vi "HFRR ADV v024 new software.vi"() -> ()   [LabVIEW 2025] (continued)
            n1309 = call "CAMERA LIVE FEED FGV.vi"("Enum - Menu"=CAMERA_LIVE_FEED_ENUM."CAMERA MINIMIZE") -> ()  [unwired: 9 in, 2 out]
          }
          frame #1 {
            n1310 = property on="Auto Scar Check  2" class="Clust (strict)"("Visible"=TRUE) -> ()  [unwired: 2 in, 2 out]
          }
          frame #2 {
            n1311 = String To Path(string="C:\\LAB-IQ\\Image Calibrate v01.dcf") -> (path=w1382:path)
            n1312 = Open/Create/Replace File ("Open File")(file path (use dialog)=w1382) -> (refnum out=w1383:refnum<file>)  [unwired: 5 in, 2 out]
            n1313 = for {
              N: 4 -> [_]
              tunnel: w1383 -> [w1389]
              i -> [w1385]
              n1314 = Read from Text File ("Read File")(file (use dialog)=w1389) -> (text=w1390:string)  [unwired: 3 in, 3 out]
              n1315 = String Subset(string=w1390, offset (0)=6, length (rest)=10 ("length (rest)")) -> (substring=w1386:string)
              n1316 = Fract/Exp String To Number(string=w1386) -> (number=w1384:dbl)  [unwired: 3 in, 1 out]
              n1317 = case shown="0" w1385 {
                tunnel: w1384 -> [w1391 w1392 _ w1393 _]
                frame 0 {
                  "5x Gain" <- w1391
                }
                frame 1 {
                  "10x Gain" <- w1392
                }
                frame 2 {
                }
                frame 3 {
                  "100x gain" <- w1393
                }
                frame 4, Default {
                }
              }
            }
          }
          frame #3 {
            n1318 = local read "FILE 3"() -> (w1399:string)
            n1319 = call <vilib>:"Trim Whitespace.vi"("string"="C:\\LAB-IQ\\images\\") -> ("trimmed string"=w1401:string)  [unwired: 1 in]
            n1320 = String To Path(string=w1401) -> (path=w1400:path)
            n1321 = Concatenate Strings(w1399, ".png" ("string")) -> (w1398:string)
            n1322 = Build Path(base path=w1400, name or relative path=w1398) -> (appended path=w1396:path)
            "Image path" <- w1396
            n1323 = Path To String(path=w1396) -> (string=w1395:string)
            n1324 = call "CAMERA LIVE FEED FGV.vi"("Enum - Menu"=CAMERA_LIVE_FEED_ENUM."CAMERA SAVE", "Image Path"=w1395) -> ()  [unwired: 8 in, 2 out]
          }
          frame #4 {
            n1325 = One Button Dialog(message="Image saved successfully") -> ()  [unwired: 1 in, 1 out]
          }
          frame #5 {
            n1326 = local read "TEST STANDARD"() -> (w1405:T3)
            n1327 = local read "Magnification len live scar"() -> (w1417:string)
            n1328 = Not(x=w1406) -> (.not. x?=w1407:bool)
            n1329 = local write "Cap Live Image"(w1407) -> ()
            n1330 = case shown="\"ISO 12156\"" w1405 {
              tunnel: ["ASTM D6079" "ISO 12156"] -> w1404
              frame "ASTM D6079", Default {
              }
              frame "ISO 12156" {
              }
            }
            n1331 = case shown="\"5x\", Default" w1417 {
              tunnel: [w1420 w1421] -> w1416
              frame "5x", Default {
                n1332 = local read "5x Gain"() -> (w1420:dbl)
              }
              frame "10x" {
                # "5x"
                n1333 = local read "10x Gain"() -> (w1421:dbl)
              }
            }
            n1334 = local read "Image path"() -> (w1415:path)
            n1335 = local read "FILE 3"() -> (w1408:string)
            n1336 = call "EDGE DETCTION.vi"("GAIN VALUE"=w1416, "Image Path"=w1415) -> ("error out"=w1414:errorcluster, "return value"=w1413:cluster{string, string, dbl, dbl, dbl})  [unwired: 8 in]
            n1337 = Bundle By Name(cluster=T25 {"File Name"="", "Test Method"="", "Operator"="", "Fuel Description"="", "Date and time"=""} ("Main Ref"), "File Name"=w1408, "Test Method"=w1404) -> (w1409:T25)
            n1338 = call "duf file read.vi"("error in (no error)"=w1414, "Main Ref"=w1409) -> ("error out"=w1412:errorcluster, "Main Ref 2"=w1410:T25)  [unwired: 8 in]
            n1339 = call "EDGE DETECTION REPORT.vi"("error in (no error)"=w1412, "return value 2"=w1413, "Main Ref"=w1410) -> ()  [unwired: 8 in, 1 out]
          }
          frame #6 {
            n1340 = property on="Auto Scar Check  2" class="Clust (strict)"("Visible"=FALSE) -> ()  [unwired: 2 in, 2 out]
          }
          frame #7 {
            n1341 = call "CAMERA LIVE FEED FGV.vi"("Enum - Menu"=CAMERA_LIVE_FEED_ENUM."CAMERA MINIMIZE", "error in (no error)"=w1425) -> ()  [unwired: 8 in, 2 out]
            n1342 = local write "Main Dashboard Buttons"(T1."Home" ("Main Dashboard Buttons")) -> ()
            n1343 = local write "Main Tab"(T2."HOME" ("Main Tab")) -> ()
          }
        }
      }
    }
    n1344 = local read "Heater Button"() -> (w1278:bool)
    n1345 = case shown="True" w1280 {
      selector: w1280 -> [_ w1555]
      frame False {
      }
      frame True {
        n1346 = Not(x=w1555) -> (.not. x?=w1553:bool)
        n1347 = local write "Frequency"(w1553) -> ()
        n1348 = local write "Tab Control 2"(T6."Frequency" ("Tab Control 2")) -> ()
      }
    }
    n1349 = case shown="True" w1279 {
      selector: w1279 -> [_ w1552]
      frame False {
      }
      frame True {
        n1350 = Not(x=w1552) -> (.not. x?=w1550:bool)
        n1351 = local write "Air Temp vs Humidity"(w1550) -> ()
        n1352 = local write "Tab Control 2"(T6."Air Temp vs Rh" ("Tab Control 2")) -> ()
      }
    }
    n1353 = case shown="True" w1281 {
      selector: w1281 -> [_ w1558]
      frame False {
      }
      frame True {
        n1354 = Not(x=w1558) -> (.not. x?=w1556:bool)
        n1355 = local write "Sample Temperature"(w1556) -> ()
        n1356 = local write "Tab Control 2"(T6."Sample Temperature" ("Tab Control 2")) -> ()
      }
    }
    n1357 = case shown="\"Custom\"" w1277 {
      frame "ASTM D6079", Default {
        w1531 = "ASTM D6079 TEST CONDITIONS" ("Standard 2")
        n1358 = local write "Standard 2"(w1531) -> ()
        n1359 = local write "Standard"(w1531) -> ()
      }
      frame "ISO 12156" {
        w1532 = "ISO 12156 TEST CONDITIONS" ("Standard 2")
        n1360 = local write "Standard 2"(w1532) -> ()
        n1361 = local write "Standard"(w1532) -> ()
      }
      frame "CEC F-096-A-06" {
        w1533 = "CEC F-096-A-06 TEST CONDITIONS" ("Standard 2")
        n1362 = local write "Standard 2"(w1533) -> ()
        n1363 = local write "Standard"(w1533) -> ()
      }
      frame "Custom" {
        w1534 = "CUSTOM TEST CONDITIONS" ("Standard 2")
        n1364 = local write "Standard 2"(w1534) -> ()
        n1365 = local write "Standard"(w1534) -> ()
      }
    }
    n1366 = case shown="True" w1278 {
      frame False {
        n1367 = local write "Temperature On Command"(TRUE ("Temperature On Command")) -> ()
        n1368 = case shown="True" "Temperature Off Command" {
          selector: "Temperature Off Command" -> [_ w1538]
          frame False {
          }
          frame True {
            n1369 = Not(x=w1538) -> (.not. x?=w1537:bool)
            n1370 = local read "EVENT LOG"() -> (w1541:string)
            n1371 = local write "Temperature Off Command"(w1537) -> ()
            n1372 = call "Event Log.vi"("Content"="Heater Off", "EVENT LOG"=w1541) -> ("EVENT LOG"=w1540:string)  [unwired: 8 in, 1 out]
            n1373 = local write "EVENT LOG"(w1540) -> ()
          }
        }
      }
      frame True {
        n1374 = local write "Temperature Off Command"(TRUE ("Temperature Off Command")) -> ()
        n1375 = case shown="True" "Temperature On Command" {
          selector: "Temperature On Command" -> [_ w1545]
          frame False {
          }
          frame True {
            n1376 = Not(x=w1545) -> (.not. x?=w1544:bool)
            n1377 = local write "Temperature On Command"(w1544) -> ()
            n1378 = disable-structure shown="Enabled" {
              disable-tunnel: "Heater On" -> [w1547 _]
              frame Enabled {
                n1379 = local read "EVENT LOG"() -> (w1548:string)
                n1380 = call "Event Log.vi"("Content"=w1547, "EVENT LOG"=w1548) -> ("EVENT LOG"=w1549:string)  [unwired: 8 in, 1 out]
                n1381 = local write "EVENT LOG"(w1549) -> ()
              }
              frame Disabled {
              }
            }
          }
        }
      }
    }
    n1382 = local read "Main Tab"() -> (w1269:T2)
    n1383 = case shown="\"About\"" w1269 {
      frame "HOME", Default {
        w1312 = T19."Enabled" ("Disabled")
        n1384 = local read "Service Password enable"() -> (w1314:bool)
        n1385 = property on="Imaging" class="Bool (strict)"("DisabledEnum"=w1312) -> ()  [unwired: 2 in, 2 out]
        n1386 = property on="Dashboard" class="Bool (strict)"("DisabledEnum"=w1312) -> ()  [unwired: 2 in, 2 out]
        n1387 = property on="Test Setup" class="Bool (strict)"("DisabledEnum"=w1312) -> ()  [unwired: 2 in, 2 out]
        n1388 = property on="Analysis" class="Bool (strict)"("DisabledEnum"=w1312) -> ()  [unwired: 2 in, 2 out]
        n1389 = property on="Home" class="Bool (strict)"("DisabledEnum"=w1312) -> ()  [unwired: 2 in, 2 out]
        n1390 = property on="Report" class="Bool (strict)"("DisabledEnum"=w1312) -> ()  [unwired: 2 in, 2 out]
        n1391 = property on="Main Dashboard Buttons" class="RadioBtnsControl (strict)"("DisabledEnum"=w1312) -> ()  [unwired: 2 in, 2 out]
        n1392 = property on="Calibration" class="Bool (strict)"("DisabledEnum"=w1312) -> ()  [unwired: 2 in, 2 out]
        n1393 = case shown="True" w1314 {
          tunnel: [T19."Disabled" ("Disabled") T19."Enabled" ("Disabled")] -> w1313
          frame False {
          }
          frame True {
          }
        }
        n1394 = property on="About" class="Bool (strict)"("DisabledEnum"=w1313) -> ()  [unwired: 2 in, 2 out]
      }
      frame "Test Setup" {
        w1319 = T19."Enabled" ("Disabled")
        n1395 = local read "Service Password enable"() -> (w1318:bool)
        n1396 = property on="Dashboard" class="Bool (strict)"("DisabledEnum"=T19."Disabled" ("Disabled")) -> ()  [unwired: 2 in, 2 out]
        n1397 = property on="Imaging" class="Bool (strict)"("DisabledEnum"=w1319) -> ()  [unwired: 2 in, 2 out]
        n1398 = property on="Analysis" class="Bool (strict)"("DisabledEnum"=w1319) -> ()  [unwired: 2 in, 2 out]
        n1399 = property on="Home" class="Bool (strict)"("DisabledEnum"=w1319) -> ()  [unwired: 2 in, 2 out]
        n1400 = property on="Report" class="Bool (strict)"("DisabledEnum"=w1319) -> ()  [unwired: 2 in, 2 out]
        n1401 = property on="Test Setup" class="Bool (strict)"("DisabledEnum"=w1319) -> ()  [unwired: 2 in, 2 out]
        n1402 = case shown="True" w1318 {
          tunnel: [T19."Disabled" ("Disabled") T19."Enabled" ("Disabled")] -> w1317
          frame False {
          }
          frame True {
          }
        }
        n1403 = property on="About" class="Bool (strict)"("DisabledEnum"=w1317) -> ()  [unwired: 2 in, 2 out]
      }
      frame "Adv Scar" {
        w1326 = T19."Enabled" ("Disabled")
        n1404 = property on="Dashboard" class="Bool (strict)"("DisabledEnum"=T19."Disabled" ("Disabled")) -> ()  [unwired: 2 in, 2 out]
        n1405 = property on="Imaging" class="Bool (strict)"("DisabledEnum"=w1326) -> ()  [unwired: 2 in, 2 out]
        n1406 = property on="Analysis" class="Bool (strict)"("DisabledEnum"=w1326) -> ()  [unwired: 2 in, 2 out]
        n1407 = property on="Home" class="Bool (strict)"("DisabledEnum"=w1326) -> ()  [unwired: 2 in, 2 out]
        n1408 = property on="Report" class="Bool (strict)"("DisabledEnum"=w1326) -> ()  [unwired: 2 in, 2 out]
        n1409 = property on="Test Setup" class="Bool (strict)"("DisabledEnum"=w1326) -> ()  [unwired: 2 in, 2 out]
        n1410 = local read "Service Password enable"() -> (w1324:bool)
        n1411 = case shown="True" w1324 {
          tunnel: [T19."Disabled" ("Disabled") T19."Enabled" ("Disabled")] -> w1323
          frame False {
          }
          frame True {
          }
        }
        n1412 = property on="About" class="Bool (strict)"("DisabledEnum"=w1323) -> ()  [unwired: 2 in, 2 out]
      }
      frame "Calibration" {
        w1329 = T19."Enabled" ("Disabled")
        n1413 = property on="Dashboard" class="Bool (strict)"("DisabledEnum"=T19."Disabled" ("Disabled")) -> ()  [unwired: 2 in, 2 out]
        n1414 = property on="Imaging" class="Bool (strict)"("DisabledEnum"=w1329) -> ()  [unwired: 2 in, 2 out]
        n1415 = property on="Analysis" class="Bool (strict)"("DisabledEnum"=w1329) -> ()  [unwired: 2 in, 2 out]
        n1416 = property on="Home" class="Bool (strict)"("DisabledEnum"=w1329) -> ()  [unwired: 2 in, 2 out]
        n1417 = property on="Report" class="Bool (strict)"("DisabledEnum"=w1329) -> ()  [unwired: 2 in, 2 out]
        n1418 = property on="Test Setup" class="Bool (strict)"("DisabledEnum"=w1329) -> ()  [unwired: 2 in, 2 out]
        n1419 = local read "Service Password enable"() -> (w1331:bool)
        n1420 = property on="Calibration" class="Bool (strict)"("DisabledEnum"=w1329) -> ()  [unwired: 2 in, 2 out]
        n1421 = case shown="True" w1331 {
          tunnel: [T19."Disabled" ("Disabled") T19."Enabled" ("Disabled")] -> w1330
          frame False {
          }
          frame True {
          }
        }
        n1422 = property on="About" class="Bool (strict)"("DisabledEnum"=w1330) -> ()  [unwired: 2 in, 2 out]
      }
      frame "Adv Scar Report" {
        w1337 = T19."Enabled" ("Disabled")
        n1423 = property on="Dashboard" class="Bool (strict)"("DisabledEnum"=T19."Disabled" ("Disabled")) -> ()  [unwired: 2 in, 2 out]
        n1424 = property on="Imaging" class="Bool (strict)"("DisabledEnum"=w1337) -> ()  [unwired: 2 in, 2 out]
        n1425 = property on="Analysis" class="Bool (strict)"("DisabledEnum"=w1337) -> ()  [unwired: 2 in, 2 out]
        n1426 = property on="Home" class="Bool (strict)"("DisabledEnum"=w1337) -> ()  [unwired: 2 in, 2 out]
        n1427 = property on="Report" class="Bool (strict)"("DisabledEnum"=w1337) -> ()  [unwired: 2 in, 2 out]
        n1428 = property on="Test Setup" class="Bool (strict)"("DisabledEnum"=w1337) -> ()  [unwired: 2 in, 2 out]
        n1429 = local read "Service Password enable"() -> (w1336:bool)
        n1430 = case shown="True" w1336 {
          tunnel: [T19."Disabled" ("Disabled") T19."Enabled" ("Disabled")] -> w1335
          frame False {
          }
          frame True {
          }
        }
        n1431 = property on="About" class="Bool (strict)"("DisabledEnum"=w1335) -> ()  [unwired: 2 in, 2 out]
      }
      frame "Compare Files" {
        w1343 = T19."Enabled" ("Disabled")
        n1432 = local read "Service Password enable"() -> (w1342:bool)
        n1433 = property on="Dashboard" class="Bool (strict)"("DisabledEnum"=T19."Disabled" ("Disabled")) -> ()  [unwired: 2 in, 2 out]
        n1434 = property on="Imaging" class="Bool (strict)"("DisabledEnum"=w1343) -> ()  [unwired: 2 in, 2 out]
        n1435 = property on="Analysis" class="Bool (strict)"("DisabledEnum"=w1343) -> ()  [unwired: 2 in, 2 out]
        n1436 = property on="Home" class="Bool (strict)"("DisabledEnum"=w1343) -> ()  [unwired: 2 in, 2 out]
        n1437 = property on="Report" class="Bool (strict)"("DisabledEnum"=w1343) -> ()  [unwired: 2 in, 2 out]
        n1438 = property on="Test Setup" class="Bool (strict)"("DisabledEnum"=w1343) -> ()  [unwired: 2 in, 2 out]
        n1439 = case shown="True" w1342 {
          tunnel: [T19."Disabled" ("Disabled") T19."Enabled" ("Disabled")] -> w1341
          frame False {
          }
          frame True {
          }
        }
        n1440 = property on="About" class="Bool (strict)"("DisabledEnum"=w1341) -> ()  [unwired: 2 in, 2 out]
      }
      frame "Acquire" {
        n1441 = local read "Service Password enable"() -> (w1348:bool)
        n1442 = property on="Test Setup" class="Bool (strict)"("DisabledEnum"=T19."Disabled" ("Disabled")) -> ()  [unwired: 2 in, 2 out]
        n1443 = local read "Auto Start Test"() -> (w1350:bool)
        n1444 = local read "RUN"() -> (w1352:bool)
        n1445 = case shown="True" w1348 {
          tunnel: [T19."Disabled" ("Disabled") T19."Enabled" ("Disabled")] -> w1349
          frame False {
          }
          frame True {
          }
        }
        n1446 = Or(x=w1352, y=w1350) -> (x .or. y?=w1351:bool)
        n1447 = case shown="True" w1351 {
          tunnel: [T19."Enabled" ("Disabled") T19."Disabled" ("Disabled")] -> w1347
          frame False {
          }
          frame True {
          }
        }
        n1448 = property on="About" class="Bool (strict)"("DisabledEnum"=w1349) -> ()  [unwired: 2 in, 2 out]
        n1449 = property on="Imaging" class="Bool (strict)"("DisabledEnum"=w1347) -> ()  [unwired: 2 in, 2 out]
        n1450 = property on="Dashboard" class="Bool (strict)"("DisabledEnum"=w1347) -> ()  [unwired: 2 in, 2 out]
        n1451 = property on="Analysis" class="Bool (strict)"("DisabledEnum"=w1347) -> ()  [unwired: 2 in, 2 out]
        n1452 = property on="Home" class="Bool (strict)"("DisabledEnum"=w1347) -> ()  [unwired: 2 in, 2 out]
        n1453 = property on="Report" class="Bool (strict)"("DisabledEnum"=w1347) -> ()  [unwired: 2 in, 2 out]
        n1454 = property on="Calibration" class="Bool (strict)"("DisabledEnum"=w1347) -> ()  [unwired: 2 in, 2 out]
      }
      frame "About" {
        n1455 = local read "FILE"() -> (w1366:string)
        n1456 = local read "TEST FILE NAM,E SAVED"() -> (w1359:bool)
        n1457 = call <vilib>:"Trim Whitespace.vi"("string"=w1366) -> ("trimmed string"=w1365:string)  [unwired: 1 in]
        n1458 = local read "Auto Start Test"() -> (w1369:bool)
        n1459 = String Length(string=w1365) -> (length=w1364:i32)
        n1460 = Greater?(x=w1364, y=1) -> (0:w1361:bool)
        n1461 = And(x=w1361, y=w1359) -> (x .and. y?=w1360:bool)
        n1462 = local read "RUN"() -> (w1371:bool)
        n1463 = case shown="True" w1360 {
          tunnel: [T19."Disabled" ("Disabled") T19."Enabled" ("Disabled")] -> w1362
          frame False {
          }
          frame True {
          }
        }
        n1464 = Or(x=w1371, y=w1369) -> (x .or. y?=w1370:bool)
        n1465 = property on="About" class="Bool (strict)"("DisabledEnum"=T19."Enabled" ("Disabled")) -> ()  [unwired: 2 in, 2 out]
        n1466 = case shown="False" w1370 {
          tunnel: [T19."Enabled" ("Disabled") T19."Disabled" ("Disabled")] -> w1368
          frame False {
          }
          frame True {
          }
        }
        n1467 = property on="Dashboard" class="Bool (strict)"("DisabledEnum"=w1362) -> ()  [unwired: 2 in, 2 out]
        n1468 = property on="Test Setup" class="Bool (strict)"("DisabledEnum"=T19."Disabled" ("Disabled")) -> ()  [unwired: 2 in, 2 out]
        n1469 = property on="Imaging" class="Bool (strict)"("DisabledEnum"=w1368) -> ()  [unwired: 2 in, 2 out]
        n1470 = property on="Analysis" class="Bool (strict)"("DisabledEnum"=w1368) -> ()  [unwired: 2 in, 2 out]
        n1471 = property on="Home" class="Bool (strict)"("DisabledEnum"=w1368) -> ()  [unwired: 2 in, 2 out]
        n1472 = property on="Report" class="Bool (strict)"("DisabledEnum"=w1368) -> ()  [unwired: 2 in, 2 out]
      }
    }
    n1473 = local read "Quit"() -> (w1296:bool)
    "Single" <- "Single - Graph"
  }
  n1474 = disable-structure shown="Disabled" {
    disable-tunnel: [w1648 _] -> w46
    disable-tunnel: _ -> [w1647 _]
    frame Disabled {
      n1475 = while {
        tunnel: w1647 -> [_]
        tunnel: [w1649] -> w1648
        tunnel: [w1650] -> _
        i -> [w1650]
        stop <- w1649 stop-if-true
        w1666 = u16 10 items=["1.0"=10, "1.5"=15, "2.0"=20] ("stop bits (10: 1 bit)")
        n1476 = Wait (ms)(milliseconds to wait=u32 10) -> ()  [unwired: 1 out]
        n1477 = call-poly "VISA Configure Serial Port"("VISA resource name"=refnum<visa-resource-name> "ASRL1::INSTR" ("COM PORT"), "timeout (10sec)"=u32 10, "baud rate (9600)"=u32 57600, "data bits (8)"=u16 8, "stop bits (10: 1 bit)"=w1666) -> ("VISA resource name out"=w1652:refnum<visa-resource-name>, "error out"=w1661:errorcluster)  [unwired: 9 in]
        n1478 = VISA Read(VISA resource name=w1652, byte count=u32 2 ("byte count (0)")) -> (read buffer=w1660:string)  [unwired: 1 in, 3 out]
        n1479 = String Subset(string=w1660, offset (0)=0, length (rest)=2 ("length (rest)")) -> (substring=w1659:string)
        n1480 = Match Pattern(string=w1659, regular expression="<>") -> (offset past match=w1656:i32)  [unwired: 1 in, 3 out]
        n1481 = Greater Or Equal?(x=w1656, y=0) -> (x >= y?=w1651:bool)
        n1482 = case shown="True" w1651 {
          tunnel: w1652 -> [_ w1670]
          tunnel: w1661 -> [_ w1669]
          frame False {
          }
          frame True {
            n1483 = VISA Read(VISA resource name=w1670, byte count=u32 32 ("byte count (0)"), error in (no error)=w1669) -> (read buffer=w1668:string)  [unwired: 3 out]
            n1484 = String Subset(string=w1668, offset (0)=0, length (rest)=8 ("length (rest)")) -> (substring=w1672:string)
            n1485 = String Subset(string=w1668, offset (0)=8, length (rest)=8 ("length (rest)")) -> (substring=w1673:string)
            n1486 = Decimal String To Number(string=w1673) -> (number=w1680:i32)  [unwired: 2 in, 1 out]
            n1487 = Decimal String To Number(string=w1672) -> (number=w1676:i32)  [unwired: 2 in, 1 out]
            n1488 = Divide(x=w1680, y=10000) -> ()  [unwired: 1 out]
            n1489 = Divide(x=w1676, y=1000000) -> ()  [unwired: 1 out]
          }
        }
        n1490 = local read "Quit"() -> (w1649:bool)
      }
    }
    frame Enabled {
    }
  }
  n1491 = Tick Count (ms)() -> (millisecond timer value=w3:u32)
  n1492 = while {
    shift-right: [w1726] -> _
    shift-left: w5 -> [w1730]
    shift-right: [w1725] -> _
    shift-left: w4 -> [w1729]
    shift-right: [w1724] -> _
    shift-left: w5 -> [w1728]
    shift-right: [w1723] -> _
    shift-left: w4 -> [w1727]
    shift-right: [w1721] -> _
    shift-left: w3 -> [w1722]
    shift-right: [w1718] -> _
    shift-left: w2 -> [w1719]
    shift-right: [w1717] -> _
    shift-left: w2 -> [w1720]
    shift-right: [w1710] -> _
    shift-left: w2 -> [w1716]
    shift-right: [w1709] -> _
    shift-left: w2 -> [w1715]
    shift-right: [w1708] -> _
    shift-left: w2 -> [w1714]
    shift-right: [w1707] -> _
    shift-left: w2 -> [w1713]
    shift-right: [w1706] -> _
    shift-left: w2 -> [w1712]
    shift-right: [w1705] -> _
    shift-left: w2 -> [w1711]
    shift-right: [w1704] -> _
    shift-left: w2 -> [w1698]
    shift-right: [w1703] -> _
    shift-left: w2 -> [w1697]
    shift-right: [w1702] -> _
    shift-left: w2 -> [w1696]
    shift-right: [w1701] -> _
    shift-left: w2 -> [w1695]
    shift-right: [w1700] -> _
    shift-left: w2 -> [w1694]
    shift-right: [w1699] -> _
    shift-left: w2 -> [w1693]
    shift-right: [w1684] -> _
    shift-left: w2 -> [w1687]
    shift-right: [w1683] -> _
    shift-left: w2 -> [w1686]
    shift-right: [w1682] -> _
    shift-left: w2 -> [w1685]
    stop <- w1732 stop-if-true
    n1493 = local read "Read UNO"() -> (w1691:string)
    n1494 = local read "Error  2"() -> (w1731:errorcluster)
    n1495 = String Length(string=w1691) -> (length=w1690:i32)
    n1496 = call <vilib>:"Trim Whitespace.vi"("string"=w1691) -> ("trimmed string"=w1692:string)  [unwired: 1 in]
    n1497 = Greater Or Equal?(x=w1690, y=23) -> (x >= y?=w1688:bool)
    n1498 = case shown="No Error" w1731 {
      tunnel: w1730 -> [w1778 w1874]
      tunnel: w1729 -> [w1777 w1873]
      tunnel: w1728 -> [w1776 w1872]
      tunnel: w1727 -> [w1775 w1871]
      tunnel: [w1774 w1874] -> w1726
      tunnel: [w1773 w1873] -> w1725
      tunnel: [w1772 w1872] -> w1724
      tunnel: [w1771 w1871] -> w1723
      tunnel: w1722 -> [w1770 w1870]
      tunnel: [w1769 w1870] -> w1721
      tunnel: w1719 -> [w1768 w1869]
      tunnel: w1720 -> [w1767 w1868]
      tunnel: [w1766 w1869] -> w1718
      tunnel: [w1765 w1868] -> w1717
      tunnel: w1716 -> [w1764 w1867]
      tunnel: w1715 -> [w1763 w1866]
      tunnel: w1714 -> [w1762 w1865]
      tunnel: w1713 -> [w1761 w1864]
      tunnel: w1712 -> [w1760 w1863]
      tunnel: w1711 -> [w1759 w1862]
      tunnel: [w1758 w1867] -> w1710
      tunnel: [w1757 w1866] -> w1709
      tunnel: [w1756 w1865] -> w1708
      tunnel: [w1755 w1864] -> w1707
      tunnel: [w1754 w1863] -> w1706
      tunnel: [w1753 w1862] -> w1705
      tunnel: w1698 -> [w1752 w1861]
      tunnel: [w1751 w1861] -> w1704
      tunnel: [w1750 w1857] -> w1703
      tunnel: [w1749 w1856] -> w1702
      tunnel: [w1748 w1860] -> w1701
      tunnel: [w1747 w1859] -> w1700
      tunnel: [w1746 w1858] -> w1699
      tunnel: w1697 -> [w1745 w1860]
      tunnel: w1696 -> [w1744 w1859]
      tunnel: w1695 -> [w1743 w1858]
      tunnel: w1694 -> [w1742 w1857]
      tunnel: w1693 -> [w1741 w1856]
      tunnel: w1692 -> [w1740 _]
      tunnel: w1688 -> [w1739 _]
      tunnel: w1687 -> [w1738 w1855]
      tunnel: w1686 -> [w1737 w1854]
      tunnel: w1685 -> [w1736 w1853]
      tunnel: [w1735 w1855] -> w1684
      tunnel: [w1734 w1854] -> w1683
      tunnel: [w1733 w1853] -> w1682
      frame No Error {
        n1499 = case shown="True" w1739 {
          tunnel: w1778 -> [w1794 w1846]
          tunnel: w1777 -> [w1793 w1845]
          tunnel: w1776 -> [w1792 w1844]
          tunnel: w1775 -> [w1791 w1843]
          tunnel: [w1794 w1842] -> w1774
          tunnel: [w1793 w1841] -> w1773
          tunnel: [w1792 w1840] -> w1772
          tunnel: [w1791 w1839] -> w1771
          tunnel: w1770 -> [w1790 w1837]
          tunnel: [w1790 w1836] -> w1769
          tunnel: w1768 -> [w1789 w1835]
          tunnel: w1767 -> [w1788 w1834]
          tunnel: [w1789 w1833] -> w1766
          tunnel: [w1788 w1832] -> w1765
          tunnel: w1764 -> [w1787 w1831]
          tunnel: w1763 -> [w1786 w1830]
          tunnel: w1762 -> [w1785 w1829]
          tunnel: w1761 -> [w1784 w1828]
          tunnel: w1760 -> [w1783 w1827]
          tunnel: w1759 -> [w1782 w1826]
          tunnel: [w1787 w1825] -> w1758
          tunnel: [w1786 w1824] -> w1757
          tunnel: [w1785 w1823] -> w1756
          tunnel: [w1784 w1822] -> w1755
          tunnel: [w1783 w1821] -> w1754
          tunnel: [w1782 w1820] -> w1753
          tunnel: w1752 -> [w1800 w1819]
          tunnel: [w1800 w1818] -> w1751
          tunnel: [w1797 w1817] -> w1750
          tunnel: [w1796 w1816] -> w1749
          tunnel: [w1799 w1815] -> w1748
          tunnel: [w1795 w1814] -> w1747
          tunnel: [w1798 w1813] -> w1746
          tunnel: w1745 -> [w1799 w1812]
          tunnel: w1744 -> [w1798 w1811]
          tunnel: w1743 -> [w1797 w1810]
          tunnel: w1742 -> [w1796 w1809]
          tunnel: w1741 -> [w1795 w1808]
          tunnel: w1740 -> [_ w1807]
          tunnel: w1738 -> [w1781 w1806]
          tunnel: w1737 -> [w1780 w1805]
          tunnel: w1736 -> [w1779 w1804]
          tunnel: [w1781 w1803] -> w1735
          tunnel: [w1780 w1802] -> w1734
          tunnel: [w1779 w1801] -> w1733
          frame False {
          }
          frame True {
            n1500 = Tick Count (ms)() -> (millisecond timer value=w1838:u32)
            n1501 = String To Byte Array(string=w1807) -> (unsigned byte array=w1851:u8[])
            n1502 = Array Size(array=w1851) -> (size(s)=w1850:i32)
            n1503 = formula code="// --- INTERNAL VARIABLE DECLARATIONS ---\nint i = 0;\nint k = 0;\nint start_idx = -1;\nint end_idx = -1;\nint phase = 0;\nint sign0 = 1;\nint sign1 = 1;\nint ch0_val = 0;   \nint ch1_val = 0;   \nfloat ch0_raw = 0.0;\nfloat ch1_raw = 0.0;\nfloat temp0 = 0.0;\nfloat temp1 = 0.0;\nfloat ch0_clean = 0.0;\nfloat ch1_clean = 0.0;\n\n// Temporal intermediate variables for calculation smoothing\nfloat raw_p2p_v = 0.0;\nfloat raw_friction = 0.0;\nfloat raw_cof = 0.0;\n\n// Initialize output variables to current shift register states right away\nout_LVDT_Min_V = in_LVDT_Min_V;\nout_LVDT_Max_V = in_LVDT_Max_V;\nout_LVDT_P2P_V = in_LVDT_P2P_V;\nout_Piezo_P2P = in_Piezo_P2P;\nout_Friction_N = in_Friction_N;\nout_COF = in_COF;\nwindow_ready = 0;\n\n// --- STEP 1: PARSE EVERY STRING IN THE BYTE ARRAY ---\nif (array_size > 2) {\n    for (i = 0; i < array_size - 1; i++) {\n        if (raw_bytes[i] == 42) { // '*' character detected\n            start_idx = i;\n        }\n        \n        // Match standard delimiter sequence \";&\" or end window character\n        if (raw_bytes[i] == 59 && raw_bytes[i+1] == 38 && start_idx != -1) { \n            end_idx = i;\n            ch0_val = 0;\n            ch1_val = 0;\n            sign0 = 1;\n            sign1 = 1;\n            phase = 0; \n\n            for (k = start_idx + 1; k < end_idx; k++) {\n                if (raw_bytes[k] == 45) { // '-' sign\n                    if (phase == 0) sign0 = -1;\n                    else sign1 = -1;\n                }\n                else if (raw_bytes[k] == 43) { // '+' sign\n                    if (phase == 0) sign0 = 1;\n                    else sign1 = 1;\n                }\n                else if (raw_bytes[k] == 59) { // ';' delimiter\n                    phase = 1; \n                }\n                else if (raw_bytes[k] >= 48 && raw_bytes[k] <= 57) { // Numeric ASCII digits\n                    if (phase == 0) {\n                        ch0_val = (ch0_val * 10) + (raw_bytes[k] - 48);\n                    } else {\n                        ch1_val = (ch1_val * 10) + (raw_bytes[k] - 48);\n                    }\n                }\n            }\n\n            // Implicit type conversion\n            ch0_raw = ch0_val * sign0 * 1.0;\n            ch1_raw = ch1_val * sign1 * 1.0;\n\n            // --- STEP 2: 3-SAMPLE MEDIAN FILTER ---\n            m0_2 = m0_1; m0_1 = m0_0; m0_0 = ch0_raw;\n            float s0_0 = m0_0; float s0_1 = m0_1; float s0_2 = m0_2;\n            if (s0_0 > s0_1) { temp0 = s0_0; s0_0 = s0_1; s0_1 = temp0; }\n            if (s0_1 > s0_2) { temp0 = s0_1; s0_1 = s0_2; s0_2 = temp0; }\n            if (s0_0 > s0_1) { temp0 = s0_0; s0_0 = s0_1; s0_1 = temp0; }\n            ch0_clean = s0_1;\n\n            m1_2 = m1_1; m1_1 = m1_0; m1_0 = ch1_raw;\n            float s1_0 = m1_0; float s1_1 = m1_1; float s1_2 = m1_2;\n            if (s1_0 > s1_1) { temp1 = s1_0; s1_0 = s1_1; s1_1 = temp1; }\n            if (s1_1 > s1_2) { temp1 = s1_1; s1_1 = s1_2; s1_2 = temp1; }\n            if (s1_0 > s1_1) { temp1 = s1_0; s1_0 = s1_1; s1_1 = temp1; }\n            ch1_clean = s1_1;\n\n            // --- STEP 3: EXPONENTIAL FILTER (STREAM LEVEL) ---\n            if (ch0_filt == 0.0) ch0_filt = ch0_clean;\n            if (ch1_filt == 0.0) ch1_filt = ch1_clean;\n\n            ch0_filt = ch0_filt + (ch0_clean - ch0_filt) * 0.125;\n            ch1_filt = ch1_filt + (ch1_clean - ch1_filt) * 0.125;\n\n            // --- STEP 4: MIN/MAX WINDOW CONTINUOUS ACCUMULATION ---\n            if (ch0_filt > max_ch0) max_ch0 = ch0_filt;\n            if (ch0_filt < min_ch0) min_ch0 = ch0_filt;\n            if (ch1_filt > max_ch1) max_ch1 = ch1_filt;\n            if (ch1_filt < min_ch1) min_ch1 = ch1_filt;\n\n            start_idx = -1; \n        }\n    }\n}\n\n// --- STEP 5: WINDOW EVALUATION ENGINE ---\nif (((current_time_ms - start_time_ms) >= 50) && (min_ch0 < 9000000.0) && (max_ch0 > -9000000.0)) {\n    window_ready = 1;\n\n    // Linear Bit-to-Voltage Transformations\n    out_LVDT_Min_V = (min_ch0 * VREF) / 8388607.0;\n    out_LVDT_Max_V = (max_ch0 * VREF) / 8388607.0;\n    raw_p2p_v = out_LVDT_Max_V - out_LVDT_Min_V;\n\n    // Piezo scaling calculations\n    out_Piezo_P2P = max_ch1 - min_ch1;\n    raw_friction = out_Piezo_P2P * PIEZO_CAL_FACTOR;\n    raw_cof = raw_friction / NORMAL_FORCE;\n\n    // --- STEP 6: OUTPUT METRIC SMOOTHING (Low-Pass Filter Alpha = 0.20) ---\n    // Seed initial historical metrics if first loop iteration\n    if (hist_LVDT_P2P == 0.0) hist_LVDT_P2P = raw_p2p_v;\n    if (hist_Friction == 0.0) hist_Friction = raw_friction;\n    if (hist_COF == 0.0)      hist_COF = raw_cof;\n\n    // Apply exponential output dampening\n    hist_LVDT_P2P = hist_LVDT_P2P + (raw_p2p_v - hist_LVDT_P2P) * 0.05;\n    hist_Friction = hist_Friction + (raw_friction - hist_Friction) * 0.05;\n    hist_COF      = hist_COF + (raw_cof - hist_COF) * 0.05;\n\n    // Direct smoothed parameters out to UI Indicators\n    out_LVDT_P2P_V = hist_LVDT_P2P;\n    out_Friction_N = hist_Friction;\n    out_COF        = hist_COF;\n\n    // Reset tracking targets to extreme boundaries safely\n    min_ch0 = 9999999.0;\n    max_ch0 = -9999999.0;\n    min_ch1 = 9999999.0;\n    max_ch1 = -9999999.0;\n\n    start_time_ms = current_time_ms;\n}"("raw_bytes"=w1851, "array_size"=w1850, "VREF"="VREF", "PIEZO_CAL_FACTOR"="PIEZO_CAL_FACTOR", "NORMAL_FORCE"="NORMAL_FORCE", "min_ch0"=w1846, "max_ch0"=w1845, "min_ch1"=w1844, "max_ch1"=w1843, "current_time_ms"=w1838, "start_time_ms"=w1837, "ch0_filt"=w1835, "ch1_filt"=w1834, "m0_0"=w1831, "m0_1"=w1830, "m0_2"=w1829, "m1_0"=w1828, "m1_1"=w1827, "m1_2"=w1826, "in_LVDT_Min_V"=w1819, "in_LVDT_Max_V"=w1812, "in_LVDT_P2P_V"=w1811, "in_Piezo_P2P"=w1810, "in_Friction_N"=w1809, "in_COF"=w1808, "hist_LVDT_P2P"=w1806, "hist_Friction"=w1805, "hist_COF"=w1804) -> ("window_ready"=→"Valid_data":dbl, "out_LVDT_Min_V"=w1818:dbl, "out_LVDT_Max_V"=w1817:dbl, "out_LVDT_P2P_V"=w1816:dbl, "out_Piezo_P2P"=w1815:dbl, "out_Friction_N"=w1814:dbl, "out_COF"=w1813:dbl, "min_ch0"=w1842:dbl, "max_ch0"=w1841:dbl, "min_ch1"=w1840:dbl, "max_ch1"=w1839:dbl, "start_time_ms"=w1836:u32, "ch0_filt"=w1833:dbl, "ch1_filt"=w1832:dbl, "m0_0"=w1825:dbl, "m0_1"=w1824:dbl, "m0_2"=w1823:dbl, "m1_0"=w1822:dbl, "m1_1"=w1821:dbl, "m1_2"=w1820:dbl, "hist_LVDT_P2P"=w1803:dbl, "hist_Friction"=w1802:dbl, "hist_COF"=w1801:dbl)
            "LVDT MIN" <- w1818
            "LVDT MAX" <- w1817
            "LVDT Peak" <- w1816
            "pizo raw" <- w1815
            "Friction" <- w1814
            "cof" <- w1813
          }
        }
      }
      frame Error {
      }
    }
    n1504 = local read "Quit"() -> (w1732:bool)
  }
  n1505 = disable-structure shown="Disabled" {
    disable-tunnel: errorcluster {"status"=TRUE, "code"=0, "source"="Init"} ("error IO") -> [w1877 _]
    disable-tunnel: [w1875 _] -> w49
    frame Disabled {
      n1506 = while {
        shift-right: [w1893] -> w1879
        shift-left: _ -> [w1884]
        shift-right: [w1892] -> w1878
        shift-left: w1877 -> [w1886]
        tunnel: [w1881] -> w1875
        tunnel: [w1891] -> _
        i -> [w1891]
        stop <- w1881 stop-if-true
        n1507 = local read "Port 1a"() -> (w1887:bool)
        n1508 = local read "Port 3"() -> (w1888:bool)
        n1509 = local read "Com Port 1"() -> (w1885:refnum<visa-resource-name>)
        n1510 = Or(x=w1888, y=w1887) -> (x .or. y?=w1890:bool)
        n1511 = Unbundle(w1886) -> ("status"=→"Port 3":bool)  [unwired: 2 out]
        n1512 = Not Equal?(x=w1885, y=w1884) -> (x != y?=w1882:bool)
        n1513 = case shown="True" w1890 {
          frame False {
            w1896 = TRUE ("Visible")
            n1514 = property on="Port 1a" class="Bool (strict)"("Visible"=w1896) -> ()  [unwired: 2 in, 2 out]
            n1515 = property on="Port 3" class="Bool (strict)"("Visible"=w1896) -> ()  [unwired: 2 in, 2 out]
          }
          frame True {
            w1897 = TRUE ("Visible")
            n1516 = property on="Port 1a" class="Bool (strict)"("Visible"=w1897) -> ()  [unwired: 2 in, 2 out]
            n1517 = property on="Port 3" class="Bool (strict)"("Visible"=w1897) -> ()  [unwired: 2 in, 2 out]
          }
        }
        n1518 = Wait (ms)(milliseconds to wait=u32 40) -> ()  [unwired: 1 out]
        n1519 = case shown="True" w1882 {
          tunnel: [w1894 errorcluster {"status"=TRUE, "code"=0, "source"="Init"} ("error out")] -> w1883
          tunnel: w1886 -> [w1894 _]
          frame False {
          }
          frame True {
          }
        }
        n1520 = case shown="No Error" w1883 {
          selector: w1883 -> [w1904 w1922]
          tunnel: [w1907 w1926] -> w1893
          tunnel: [w1906 w1920] -> w1892
          tunnel: w1884 -> [w1905 w1924]
          frame No Error {
            n1521 = property class="Instr"(reference=w1905, error in=w1904) -> (reference out=w1902:refnum<visa-resource-name>, error out=w1903:errorcluster, "Serial Settings:Number of Bytes at Serial Port"=w1899:u32)
            n1522 = Greater?(x=w1899, y=u32 5) -> (0:w1898:bool)
            n1523 = Not(x=w1898) -> (.not. x?=→"Port 1a":bool)
            n1524 = while {
              tunnel: [w1915] -> w1906
              tunnel: [w1914] -> w1907
              tunnel: w1903 -> [w1913]
              tunnel: w1902 -> [w1912]
              stop <- TRUE stop-if-true
              n1525 = property class="Instr" props=["Serial Settings:Number of Bytes at Serial Port"](reference=w1912, error in=w1913) -> (reference out=w1917:refnum<visa-resource-name>, error out=w1916:errorcluster)  [unwired: 1 out]
              n1526 = VISA Read(VISA resource name=w1917, byte count=u32 50, error in (no error)=w1916) -> (VISA resource name out=w1914:refnum<visa-resource-name>, read buffer=w1909:string, error out=w1915:errorcluster)  [unwired: 1 out]
              n1527 = Wait (ms)(milliseconds to wait=u32 5) -> ()  [unwired: 1 out]
            }
          }
          frame Error {
            w1932 = u16 0 items=["None", "XON/XOFF", "RTS/CTS", "XON/XOFF & RTS/CTS", "DTR/DSR", "XON/XOFF & DTR/DSR"] ("flow control (0:none)  2")
            w1930 = u16 10 items=["1.0"=10, "1.5"=15, "2.0"=20] ("stop bits 2")
            w1928 = u16 0 items=["None", "Odd", "Even", "Mark", "Space"] ("parity 2")
            w1929 = u32 10000  # timeout (10sec)
            n1528 = VISA Close(VISA resource name=w1924, error in (no error)=w1922) -> (error out=w1925:errorcluster)
            n1529 = local write "Port 1a"(FALSE ("Port 1a")) -> ()
            n1530 = local read "Com Port 1"() -> (w1919:refnum<visa-resource-name>)
            n1531 = call <vilib>:"Clear Errors.vi"("error in (no error)"=w1925) -> ("error out"=w1923:errorcluster)  [unwired: 5 in, 1 out]
            n1532 = call-poly "VISA Configure Serial Port"("VISA resource name"=w1919, "timeout (10sec)"=w1929, "baud rate (9600)"=u32 250000 ("baud rate  2"), "data bits (8)"=u16 8 ("data bits  2"), "parity (0:none)"=w1928, "error in (no error)"=w1923, "stop bits (10: 1 bit)"=w1930, "flow control (0:none)"=w1932) -> ("VISA resource name out"=w1933:refnum<visa-resource-name>, "error out"=w1934:errorcluster)  [unwired: 6 in]
            n1533 = flat-sequence {
              tunnel: w1933 -> [w1936]
              tunnel: w1934 -> [w1935]
              tunnel: [w1936] -> w1926
              tunnel: [w1935] -> w1920
              frame #0 {
                n1534 = Wait (ms)(milliseconds to wait=u32 50) -> ()  [unwired: 1 out]
              }
            }
            "Residual Uno" <- ""
            "Port 1 Error" <- w1920
          }
        }
        n1535 = local read "Quit"() -> (w1881:bool)
        "Error Uno" <- w1886
      }
      n1536 = VISA Close(VISA resource name=w1879, error in (no error)=w1878) -> (error out=w1876:errorcluster)
      n1537 = call <vilib>:"Clear Errors.vi"("error in (no error)"=w1876) -> ()  [unwired: 5 in, 2 out]
    }
    frame Enabled {
    }
  }
  n1538 = while {
    stop <- w1947 stop-if-true
    # "V0OLTAGE TO STROKE (peice vise calibration)"
    n1539 = local read "LVDT MIN"() -> (w1939:dbl)
    n1540 = local read "LVDT Peak"() -> (w1938:dbl)
    n1541 = Wait (ms)(milliseconds to wait=u32 10) -> ()  [unwired: 1 out]
    n1542 = formula code="// Dynamic Parameterized Linear Interpolation Node\n// Inputs: vpp_val, voltages (Array), distances (Array)\n// Outputs: stroke\n\nint i = 0;\nint segments = 11; // 12 points make 11 interpolation segments\n\n// 1. Lower Boundary Clamp\nif (vpp_val <= voltages[0]) {\n    stroke = distances[0];\n}\n// 2. Upper Boundary Clamp\nelse if (vpp_val >= voltages[segments]) {\n    stroke = distances[segments];\n}\n// 3. Dynamic Segment Search Loop\nelse {\n    stroke = distances[0]; // Fallback baseline\n    for (i = 0; i < segments; i++) {\n        if (vpp_val >= voltages[i] && vpp_val <= voltages[i+1]) {\n            // Standard linear interpolation formula using array lookups\n            stroke = distances[i] + (vpp_val - voltages[i]) * (distances[i+1] - distances[i]) / (voltages[i+1] - voltages[i]);\n            break; // Segment found, safely exit the loop\n        }\n    }\n}"("vpp_val"=w1938, "voltages"="calibration values", "distances"="STROKE") -> ("stroke"=→"LVDT STROKE":dbl)
    n1543 = local read "Calibration Tare Value"() -> (w1943:dbl)
    n1544 = local read "Calibration Tare"() -> (w1941:bool)
    n1545 = Subtract(x=w1939, y=w1943) -> (x-y=→"LVDT STROKE  Calibration":dbl)
    n1546 = case shown="True" w1941 {
      selector: w1941 -> [_ w1949]
      tunnel: w1939 -> [_ w1950]
      frame False {
      }
      frame True {
        n1547 = Not(x=w1949) -> (.not. x?=w1948:bool)
        n1548 = local write "Calibration Tare"(w1948) -> ()
        "Calibration Tare Value" <- w1950
      }
    }
    n1549 = local read "Quit"() -> (w1947:bool)
  }
  n1550 = while {
    stop <- w1970 stop-if-true
    n1551 = call <vilib>:"High Resolution Polling Wait.vi"("seconds to wait"=0.02) -> ()  [unwired: 10 in, 1 out]
    n1552 = local read "Due read"() -> (w1968:string)
    n1553 = Spreadsheet String To Array(delimiter (Tab)=";", format string="", spreadsheet string=w1968, array type (2D Dbl)=string[] []) -> (array=w1965:string[])
    n1554 = Fract/Exp String To Number(string=w1965) -> (number=w1964:dbl[])  [unwired: 3 in, 1 out]
    n1555 = Index Array(array=w1964) -> (element #1=→"Sample Temperature":dbl, element #2=→"Target Sample Temperature":dbl, element #3=→"Current Duty Cycle":dbl, element #4=→"Ambient Temperature":dbl, element #5=→"Dac Status":dbl, element #6=→"Vpp":dbl, element #7=→"Active Error Code":dbl, element #8=→"Kp":dbl, element #9=→"Ki":dbl, element #10=→"Kd":dbl, element #11=→"SampleRaw":dbl, element #12=→"AmbRaw":dbl)  [unwired: 12 in]
    n1556 = local read "Quit"() -> (w1970:bool)
  }
  n1557 = while {
    shift-right: [w1984] -> w44
    shift-left: _ -> [w1976]
    shift-right: [w1971] -> w43
    shift-left: errorcluster {"status"=FALSE, "code"=0, "source"="Init"} ("error out") -> [w1978]
    tunnel: [w1973] -> w48
    tunnel: [w1983] -> _
    i -> [w1983]
    stop <- w1973 stop-if-true
    n1558 = local read "Com Port 2"() -> (w1977:refnum<visa-resource-name>)
    n1559 = local read "Port 2a"() -> (w1979:bool)
    n1560 = Unbundle(w1978) -> ("status"=→"Port 4":bool)  [unwired: 2 out]
    n1561 = call <vilib>:"High Resolution Polling Wait.vi"("seconds to wait"=0.02) -> ()  [unwired: 10 in, 1 out]
    n1562 = local read "Port 4"() -> (w1980:bool)
    n1563 = Not Equal?(x=w1977, y=w1976) -> (x != y?=w1975:bool)
    n1564 = Or(x=w1980, y=w1979) -> (x .or. y?=w1982:bool)
    n1565 = case shown="False" w1982 {
      frame False {
        w1987 = TRUE ("Visible")
        n1566 = property on="Port 2a" class="Bool (strict)"("Visible"=w1987) -> ()  [unwired: 2 in, 2 out]
        n1567 = property on="Port 4" class="Bool (strict)"("Visible"=w1987) -> ()  [unwired: 2 in, 2 out]
      }
      frame True {
        w1988 = TRUE ("Visible")
        n1568 = property on="Port 2a" class="Bool (strict)"("Visible"=w1988) -> ()  [unwired: 2 in, 2 out]
        n1569 = property on="Port 4" class="Bool (strict)"("Visible"=w1988) -> ()  [unwired: 2 in, 2 out]
      }
    }
    n1570 = case shown="True" w1975 {
      tunnel: [w1985 errorcluster {"status"=TRUE, "code"=0, "source"="Init"} ("error out")] -> w1974
      tunnel: w1978 -> [w1985 _]
      frame False {
      }
      frame True {
      }
    }
    n1571 = case shown="No Error" w1974 {
      selector: w1974 -> [w2001 w2032]
      tunnel: [w1994 w2037] -> w1984
      tunnel: [w2002 w2030] -> w1971
      tunnel: w1976 -> [w2003 w2035]
      frame No Error {
        n1572 = property class="Instr" props=["Serial Settings:Number of Bytes at Serial Port"](reference=w2003, error in=w2001) -> (reference out=w1995:refnum<visa-resource-name>, error out=w2000:errorcluster)  [unwired: 1 out]
        n1573 = while {
          tunnel: [w2011] -> w1996
          tunnel: [w2010] -> w1997
          tunnel: w2000 -> [w2009]
          tunnel: w1995 -> [w2008]
          tunnel: [w2007] -> _
          i -> [w2007]
          stop <- TRUE stop-if-true
          n1574 = property class="Instr" props=["Serial Settings:Number of Bytes at Serial Port"](reference=w2008, error in=w2009) -> (reference out=w2013:refnum<visa-resource-name>, error out=w2012:errorcluster)  [unwired: 1 out]
          n1575 = VISA Read(VISA resource name=w2013, byte count=u32 1000, error in (no error)=w2012) -> (VISA resource name out=w2010:refnum<visa-resource-name>, read buffer=→"Due read":string, error out=w2011:errorcluster)  [unwired: 1 out]
        }
        n1576 = local read "Due Write"() -> (w1993:string)
        n1577 = call <vilib>:"Trim Whitespace.vi"("string"=w1993) -> ("trimmed string"=w1992:string)  [unwired: 1 in]
        n1578 = Not Equal?(x=w1992, y="") -> (x != y?=w1998:bool)
        n1579 = VISA Flush I/O Buffer(VISA resource name=w1997) -> (VISA resource name out=w1990:refnum<visa-resource-name>, error out=→"error out 10":errorcluster)  [unwired: 2 in]
        n1580 = case shown="True" w1998 {
          tunnel: w1990 -> [w2015 w2020]
          tunnel: [w2015 w2024] -> w1994
          tunnel: w1996 -> [w2014 w2019]
          tunnel: [w2014 w2022] -> w2002
          tunnel: w1992 -> [_ w2018]
          tunnel: [_ w2021] -> _
          frame False {
            # "DATA  WRITE LOOP"
          }
          frame True {
            n1581 = Concatenate Strings(w2018, "\r\n") -> (w2017:string)
            n1582 = VISA Write(VISA resource name=w2020, write buffer=w2017, error in (no error)=w2019) -> (VISA resource name out=w2024:refnum<visa-resource-name>, return count=w2021:u32, error out=w2023:errorcluster)
            n1583 = flat-sequence {
              tunnel: w2023 -> [w2026]
              tunnel: [w2026] -> w2022
              frame #0 {
                n1584 = local write "Due Write"("" ("Command")) -> ()
                n1585 = Wait (ms)(milliseconds to wait=u32 5) -> ()  [unwired: 1 out]
              }
            }
          }
        }
        "Port 2a" <- TRUE ("Port 2a")
      }
      frame Error {
        w2043 = u16 0 items=["None", "XON/XOFF", "RTS/CTS", "XON/XOFF & RTS/CTS", "DTR/DSR", "XON/XOFF & DTR/DSR"] ("flow control (0:none)  2")
        w2041 = u16 10 items=["1.0"=10, "1.5"=15, "2.0"=20] ("stop bits 2")
        w2039 = u16 0 items=["None", "Odd", "Even", "Mark", "Space"] ("parity 2")
        w2040 = u32 10000  # timeout (10sec)
        n1586 = VISA Clear(VISA resource name=w2035, error in (no error)=w2032) -> (VISA resource name out=w2034:refnum<visa-resource-name>, error out=w2033:errorcluster)
        n1587 = VISA Close(VISA resource name=w2034, error in (no error)=w2033) -> (error out=w2036:errorcluster)
        n1588 = call <vilib>:"Clear Errors.vi"("error in (no error)"=w2036) -> ()  [unwired: 5 in, 2 out]
        n1589 = local write "Port 2a"(FALSE ("Port 2a")) -> ()
        n1590 = local read "Com Port 2"() -> (w2029:refnum<visa-resource-name>)
        "visa due" <- w2029
        n1591 = call-poly "VISA Configure Serial Port"("VISA resource name"=w2029, "timeout (10sec)"=w2040, "baud rate (9600)"=u32 250000 ("baud rate  2"), "data bits (8)"=u16 8 ("data bits  2"), "parity (0:none)"=w2039, "stop bits (10: 1 bit)"=w2041, "flow control (0:none)"=w2043) -> ("VISA resource name out"=w2044:refnum<visa-resource-name>, "error out"=w2045:errorcluster)  [unwired: 7 in]
        n1592 = flat-sequence {
          tunnel: w2044 -> [w2047]
          tunnel: w2045 -> [w2046]
          tunnel: [w2047] -> w2037
          tunnel: [w2046] -> w2030
          frame #0 {
            n1593 = Wait (ms)(milliseconds to wait=u32 50) -> ()  [unwired: 1 out]
          }
        }
        "Residual Due" <- ""
        "Port 2 Error" <- w2030
      }
    }
    "error out 9" <- w1971
    n1594 = local read "Quit"() -> (w1973:bool)
    "Error Due" <- w1978
  }
  n1595 = local write "FRICVALZ"(0.0 ("FRICVALZ")) -> ()
  n1596 = property on="RUN" class="Bool (strict)"("Visible"=TRUE) -> ()  [unwired: 2 in, 2 out]
  n1597 = while {
    tunnel: [w2064] -> _
    tunnel: [w2049] -> w58
    i -> [w2064]
    stop <- w2049 stop-if-true
    n1598 = local read "conststatus"() -> (w2053:dbl)
    n1599 = local read "Main Tab"() -> (w2051:T2)
    n1600 = local read "EDIT"() -> (w2070:bool)
    n1601 = local read "Rate"() -> (w2069:dbl)
    n1602 = case shown="True" w2070 {
      tunnel: [FALSE TRUE] -> w2056
      frame False {
      }
      frame True {
      }
    }
    n1603 = property on="Time slide" class="Slide (strict)"("Scale.Range:Maximum"=2500.0) -> ()  [unwired: 2 in, 2 out]
    n1604 = Equal?(x=w2051, y=T27."About" ("Main Tab")) -> (x = y?=w2062:bool)
    n1605 = Equal?(x=w2053, y=0.0) -> (x = y?=w2054:bool)
    n1606 = Divide(x=1.0, y=w2069) -> (x/y=w2065:dbl)
    "Time 2" <- w2065
    n1607 = case shown="True" w2054 {
      frame False {
      }
      frame True {
        # "C:\\WinDucom\\calibrate WO 2391.dcf"
        n1608 = local write "Lan flag"(22) -> ()
        n1609 = local write "conststatus"(10.0 ("rpm value : 2")) -> ()
        n1610 = String To Path(string="C:\\LAB-IQ\\calibrate WO 2465.dcf") -> (path=w2076:path)
        n1611 = Open/Create/Replace File "Open File"(file path (use dialog)=w2076) -> (refnum out=w2074:refnum<file>)  [unwired: 5 in, 2 out]
        n1612 = for {
          N: 23 -> [_]
          tunnel: w2074 -> [w2085]
          i -> [w2079]
          (unwired) TRUE ("line mode (F)")
          n1613 = Read from Text File "Read File"(file (use dialog)=w2085) -> (text=w2084:string)  [unwired: 3 in, 3 out]
          n1614 = Match Pattern(string=w2084, regular expression="]") -> (after substring=w2082:string)  [unwired: 1 in, 3 out]
          n1615 = String Subset(string=w2084, offset (0)=5, length (rest)=10 ("length (rest)")) -> (substring=w2077:string)
          n1616 = Fract/Exp String To Number(string=w2077) -> (number=w2078:dbl)  [unwired: 3 in, 1 out]
          n1617 = Match Pattern(string=w2082, regular expression="-") -> (before substring=w2080:string)  [unwired: 1 in, 3 out]
          n1618 = case shown="15" w2079 {
            tunnel: w2078 -> [w2088 w2089 w2090 w2091 _ _ _ w2096 w2097 _ w2098 _ _ _ _ _ _ w2099 w2100 _ _ _ _ _]
            tunnel: w2080 -> [_ _ _ _ w2092 w2093 w2094 _ _ _ _ _ _ _ _ _ _ _ _ w2101 w2102 w2103 w2104 _]
            frame 0 {
              n1619 = local write "FRIC. FORCE :"(w2088) -> ()
            }
            frame 1 {
              n1620 = local write "TEMPERATURE :"(w2089) -> ()
            }
            frame 2 {
              n1621 = local write "HUMIDITY:"(w2090) -> ()
            }
            frame 3 {
              n1622 = local write "AIR TEMPERATURE :"(w2091) -> ()
            }
            frame 4 {
              n1623 = local write "Com Port 1"(w2092) -> ()
            }
            frame 5 {
              n1624 = local write "Com Port 2"(w2093) -> ()
              n1625 = local write "visa due"(w2093) -> ()
            }
            frame 6 {
              n1626 = String To Path(string=w2094) -> (path=w2095:path)
              n1627 = local write "File Path"(w2095) -> ()
              "String" <- w2094
            }
            frame 7 {
              n1628 = local write "DISPLACEMENT :"(w2096) -> ()
            }
            frame 8 {
              n1629 = local write "STROKE GAIN :"(w2097) -> ()
            }
            frame 9 {
            }
            frame 10 {
              n1630 = local write "Language Selection"(w2098) -> ()
            }
            frame 11 {
            }
            frame 12 {
            }
            frame 13 {
            }
            frame 14 {
            }
            frame 15 {
            }
            frame 16 {
            }
            frame 17 {
              n1631 = local write "AIR TEMP INTERCEPT:"(w2099) -> ()
            }
            frame 18 {
              n1632 = local write "TEMP INTERCEPT:"(w2100) -> ()
            }
            frame 21 {
              n1633 = local write "S.NO"(w2101) -> ()
            }
            frame 22 {
              n1634 = local write "Com Port 3"(w2102) -> ()
            }
            frame 20 {
              n1635 = local write "Camera Port :"(w2103) -> ()
            }
            frame 19 {
              n1636 = local write "C3 :"(w2104) -> ()
            }
            frame 23, Default {
            }
          }
        }
      }
    }
    n1637 = Select(t=u32 2500 ("milliseconds to wait"), s=w2062, f=u32 500 ("milliseconds to wait")) -> (s? t:f=w2060:u32)
    n1638 = Multiply(x=w2065, y=w2060) -> (x*y=w2067:dbl)
    n1639 = property on="Time slide" class="Slide (strict)"("Visible"=w2056) -> ()  [unwired: 2 in, 2 out]
    n1640 = call "Elapsed Time2"("Time Target (s)"=w2067, "Auto Reset"=TRUE) -> ("Time has Elapsed"=w2057:bool)  [unwired: 10 in, 7 out]
    n1641 = case shown="True" w2057 {
      frame False {
      }
      frame True {
        n1642 = stacked-sequence {
          frame #0 {
            # "DATA PROCESSING"
            # "115 mV/N"
            n1643 = local read "Sample Temperature"() -> (w2107:dbl)
            n1644 = local read "RH Numeric:"() -> (w2114:dbl)
            n1645 = local read "HUMIDITY:"() -> (w2115:dbl)
            n1646 = local read "FRICVALZ"() -> (w2126:dbl)
            n1647 = local read "Friction"() -> (w2110:dbl)
            n1648 = Multiply(x=w2114, y=w2115) -> (x*y=→"Humidity ( %RH )" →"Hum" →"Hum 2":dbl)
            n1649 = call <vilib>:"Mean PtByPt.vi"("x"=w2107, "sample length"=100) -> ("mean"=w2106:dbl)  [unwired: 2 in, 1 out]
            "TEMP 2" <- w2106
            "TEMP 3" <- w2106
            n1650 = Subtract(x=w2110, y=w2126) -> (x-y=w2121:dbl)
            "FF 2" <- w2121
            "FF 4" <- w2121
            n1651 = local read "Ambient Temperature"() -> (→"AIR TEMP":dbl)
            n1652 = local read "TEMP"() -> (w2125:dbl)
            n1653 = local write "FF 3"(w2121) -> ()
            n1654 = Compound Arithmetic op=OR("FRICVALZ 4", "FRICVALZ 3", "FRICVALZ 2") -> (w2117:bool)
            n1655 = case shown="True" w2117 {
              tunnel: w2110 -> [_ w2132]
              frame False {
              }
              frame True {
                w2131 = FALSE ("FRICVALZ")
                n1656 = local write "FRICVALZ 3"(w2131) -> ()
                n1657 = local write "FRICVALZ 2"(w2131) -> ()
                n1658 = local write "FRICVALZ 4"(w2131) -> ()
                "FRICVALZ" <- w2132
              }
            }
            n1659 = Not A Number/Path/Refnum?(number/path/refnum=w2125) -> (NaN/Path/Refnum?=w2124:bool)
            n1660 = Not A Number/Path/Refnum?(number/path/refnum=w2121) -> (NaN/Path/Refnum?=w2123:bool)
            n1661 = Divide(x=w2121, y=1.96) -> (x/y=w2118:dbl)
            n1662 = Compound Arithmetic op=OR(w2124, w2123) -> (w2122:bool)
            n1663 = Not A Number/Path/Refnum?(number/path/refnum=w2118) -> (NaN/Path/Refnum?=w2119:bool)
            n1664 = case shown="True" w2122 {
              frame False {
              }
              frame True {
                n1665 = local write "TEMP"(0.0 ("TEMP")) -> ()
                n1666 = local write "FF 2"(0.0 ("FF 2")) -> ()
                n1667 = local write "reinit"(TRUE ("reinit")) -> ()
              }
            }
            n1668 = local write "TEMP"(w2106) -> ()
            n1669 = Select(t=0.0, s=w2119, f=w2118) -> (s? t:f=w2109:dbl)
            "COF 2" <- w2109
            n1670 = local write "COF 3"(w2109) -> ()
          }
        }
      }
    }
    n1671 = Wait (ms)(milliseconds to wait=u32 50) -> ()  [unwired: 1 out]
    n1672 = local read "Quit"() -> (w2049:bool)
    "Rate" <- 2500.0 ("No of Samples")
  }
  n1673 = while {
    tunnel: w61 -> [_]
